vi "Display_Seconds.vi"(7 "Enum":T1, 8 "error in (no error)":errorcluster, 10 "Display In":string, 11 "Time (s) In":dbl) -> (0 "error out":errorcluster, 2 "Time (s) Out":dbl, 3 "Display Out":string)   [LabVIEW 2026]
uses:
  controls/Time and Display Conversion.ctl
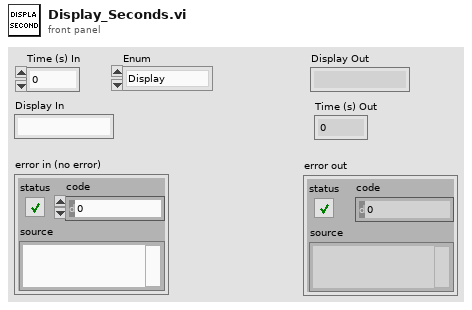
[diagram p1: front panel]
types:
  T1 = typedef "Time and Display Conversion.ctl" = enum16{"Display", "Time (s)"}
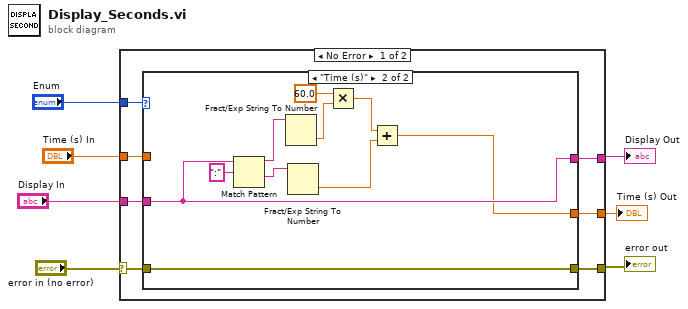
[diagram p0: block diagram]
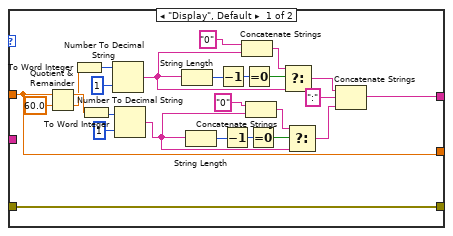
[diagram p2: hidden frame]
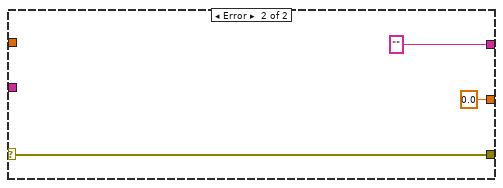
[diagram p3: hidden frame]
diagram:
  n1 = case shown="No Error" "error in (no error)" {
    selector: "error in (no error)" -> [w11 w52]
    tunnel: "Time (s) In" -> [w14 _]
    tunnel: [w13 ""] -> w6
    tunnel: [w10 w52] -> w4
    tunnel: "Enum" -> [w12 _]
    tunnel: "Display In" -> [w9 _]
    tunnel: [w8 0.0 ("Time (s) In")] -> w1
    frame No Error {
      n2 = case shown="\"Time (s)\"" w12 {
        tunnel: w14 -> [w15 _]
        tunnel: [w19 w48] -> w13
        tunnel: w11 -> [w16 w49]
        tunnel: [w16 w49] -> w10
        tunnel: w9 -> [_ w48]
        tunnel: [w15 w40] -> w8
        frame "Display", Default {
          n3 = Quotient & Remainder(x=w15, y=60.0) -> (x-y*floor(x/y)=w23:dbl, floor(x/y)=w21:dbl)
          n4 = To Word Integer(number=w21) -> (16bit integer=w22:i16)
          n5 = To Word Integer(number=w23) -> (16bit integer=w24:i16)
          n6 = Number To Decimal String(number=w22, width (-)=i16 1 ("precision (6)")) -> (decimal integer string=w31:string)
          n7 = Number To Decimal String(number=w24, width (-)=i16 1) -> (decimal integer string=w37:string)
          n8 = String Length(string=w31) -> (length=w27:i32)
          n9 = String Length(string=w37) -> (length=w34:i32)
          n10 = Decrement(x=w27) -> (x-1=w26:i32)
          n11 = Decrement(x=w34) -> (x-1=w33:i32)
          n12 = Concatenate Strings("0" ("string"), w31) -> (w30:string)
          n13 = Equal To 0?(x=w26) -> (x = 0?=w28:bool)
          n14 = Concatenate Strings("0" ("string"), w37) -> (w36:string)
          n15 = Equal To 0?(x=w33) -> (x = 0?=w35:bool)
          n16 = Select(t=w30, s=w28, f=w31) -> (s? t:f=w32:string)
          n17 = Select(t=w36, s=w35, f=w37) -> (s? t:f=w39:string)
          n18 = Concatenate Strings(w32, ":" ("string"), w39) -> (w19:string)
        }
        frame "Time (s)" {
          n19 = Match Pattern(string=w48, regular expression=":") -> (before substring=w46:string, after substring=w42:string)  [unwired: 1 in, 2 out]
          n20 = Fract/Exp String To Number(string=w46) -> (number=w44:dbl)  [unwired: 3 in, 1 out]
          n21 = Fract/Exp String To Number(string=w42) -> (number=w41:dbl)  [unwired: 3 in, 1 out]
          n22 = Multiply(x=60.0, y=w44) -> (x*y=w43:dbl)
          n23 = Add(x=w43, y=w41) -> (x+y=w40:dbl)
        }
      }
    }
    frame Error {
    }
  }
  "Display Out" <- w6
  "error out" <- w4
  "Time (s) Out" <- w1
